vi "Digitizer Clock In Data.vi"(6 "Digitize Read Delay Ticks":u32, 9 "Digitize # Bits":u32=16, 10 "Convert Clock Ticks":u32=20, 11 "Refnum in":refnum<k21>) -> (3 "Data Out":T1 format="%.0x")   [LabVIEW 2017]
doc: "Author: Scott Hannahs <sth@magnet.fsu.edu>\nCopyright 2018 Florida State University, All rights reserved."
uses:
  <vilib>/eio/EIONode/EIONode.xnode
  <vilib>/rvi/eio/common/nirviEmuTemplateMethod_errors.vi
  SCH Data Controls/SCH Raw Int Data.ctl
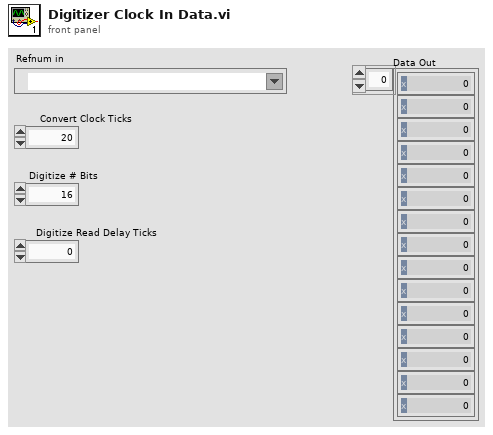
[diagram p1: front panel]
types:
  T1 = typedef "SCH Raw Int Data.ctl" = i16[]
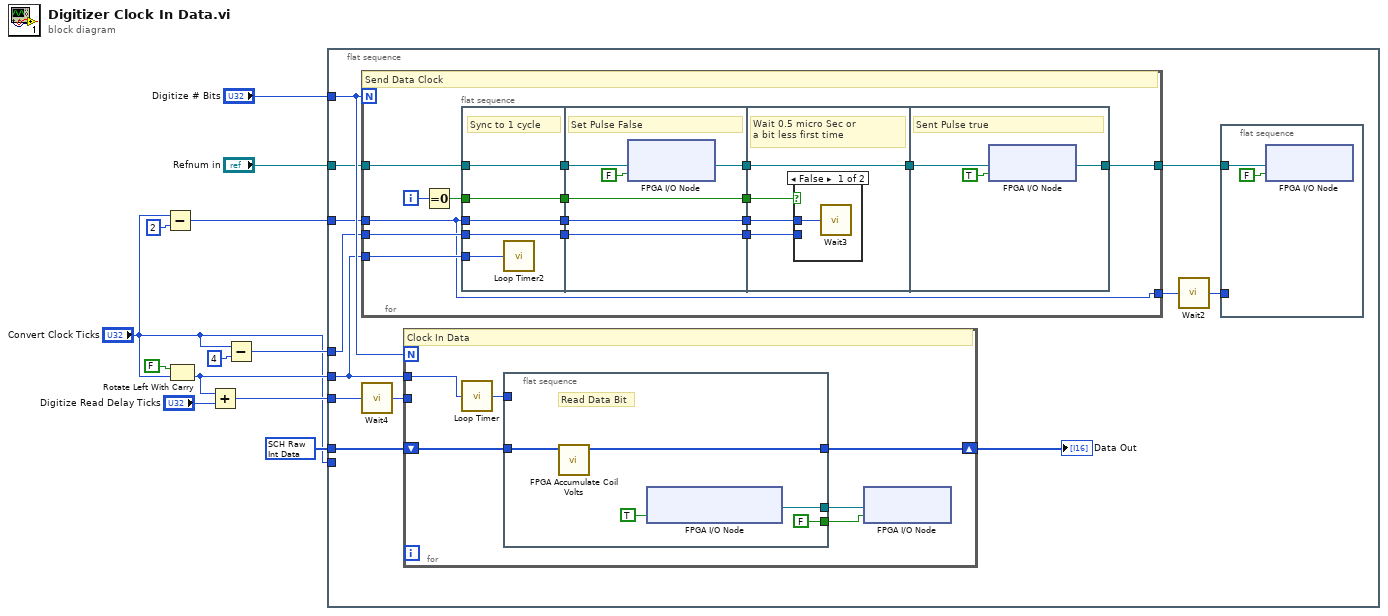
[diagram p0: block diagram]
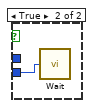
[diagram p2: hidden frame]
diagram:
  n1 = Subtract(x="Convert Clock Ticks", y=u32 2) -> (x-y=w1:u32)
  n2 = Rotate Left With Carry(2:"Convert Clock Ticks", 3:FALSE ("carry")) -> (0:w4:u32)  [unwired: 1 out]
  n3 = Add(x=w4, y="Digitize Read Delay Ticks") -> (x+y=w6:u32)
  n4 = Subtract(x="Convert Clock Ticks", y=u32 4) -> (x-y=w7:u32)
  n5 = flat-sequence {
    tunnel: "Digitize # Bits" -> [w24]
    tunnel: "Convert Clock Ticks" -> [_]
    tunnel: T1 [0, 0, 0, 0, 0, 0, 0, 0, 0, 0, 0, 0, 0, 0, 0, 0, 0, 0, 0, 0, 0, 0, 0, 0, 0, 0, 0, 0, 0, 0, 0, 0, 0, 0, 0, 0, 0, 0] -> [w22]
    tunnel: "Refnum in" -> [w21]
    tunnel: w4 -> [w20]
    tunnel: w7 -> [w19]
    tunnel: w6 -> [w18]
    tunnel: w1 -> [w17]
    frame #0 {
      n6 = for {
        N: w24 -> [_]
        tunnel: w21 -> [w42]
        tunnel: w20 -> [w39]
        tunnel: w19 -> [w37]
        tunnel: [w28] -> w15
        tunnel: [w27] -> w14
        tunnel: w17 -> [w27]
        i -> [w41]
        # "Send Data Clock"
        n7 = Equal To 0?(x=w41) -> (x = 0?=w38:bool)
        n8 = flat-sequence {
          tunnel: w37 -> [w44]
          tunnel: w38 -> [w45]
          tunnel: w39 -> [w43]
          tunnel: w27 -> [w46]
          tunnel: w42 -> [w47]
          tunnel: [w47] -> w36
          tunnel: [w46] -> w34
          tunnel: [w45] -> w32
          tunnel: [w44] -> w30
          tunnel: w36 -> [w50]
          tunnel: [w49] -> w35
          tunnel: w34 -> [w53]
          tunnel: [w53] -> w33
          tunnel: w32 -> [w52]
          tunnel: [w52] -> w31
          tunnel: w30 -> [w51]
          tunnel: [w51] -> w29
          tunnel: [w57] -> w40
          tunnel: w35 -> [w57]
          tunnel: w33 -> [w54]
          tunnel: w31 -> [w56]
          tunnel: w29 -> [w55]
          tunnel: w40 -> [w61]
          tunnel: [w60] -> w28
          frame #0 {
            # "Sync to 1 cycle"
            n9 = call "Loop Timer2"("Count(Ticks)"=w43) -> ()  [unwired: 1 out]
          }
          frame #1 {
            # "Set Pulse False"
            n10 = xnode "FPGA I/O Node"("I/O Item"=FALSE, "FPGA I/O In"=w50) -> ("FPGA I/O Out"=w49:refnum<k21>)  [unwired: 1 in, 1 out]
          }
          frame #2 {
            # "Wait 0.5 micro Sec or\na bit less first time"
            n11 = case shown="False" w56 {
              tunnel: w55 -> [_ w59]
              tunnel: w54 -> [w58 _]
              frame False {
                n12 = call "Wait3"("Count(Ticks)"=w58) -> ()  [unwired: 1 out]
              }
              frame True {
                n13 = call "Wait"("Count(Ticks)"=w59) -> ()  [unwired: 1 out]
              }
            }
          }
          frame #3 {
            # "Sent Pulse true"
            n14 = xnode "FPGA I/O Node"("I/O Item"=TRUE ("Connector0/DIO0"), "FPGA I/O In"=w61) -> ("FPGA I/O Out"=w60:refnum<k21>)
          }
        }
      }
      n15 = call "Wait4"("Count(Ticks)"=w18) -> ("Tick Count(Ticks)"=w23:u32)
      n16 = for {
        N: w24 -> [_]
        shift-right: [w68] -> w16
        shift-left: w22 -> [w67]
        tunnel: w23 -> [_]
        tunnel: w20 -> [w65]
        # "Clock In Data"
        n17 = call "Loop Timer"("Count(Ticks)"=w65) -> ("Tick Count(Ticks)"=w66:u32)
        n18 = flat-sequence {
          tunnel: [w73] -> w68
          tunnel: w67 -> [w72]
          tunnel: w66 -> [_]
          tunnel: [FALSE ("Digizer Data Read")] -> w64
          tunnel: [w69] -> w63
          frame #0 {
            # "Read Data Bit"
            n19 = call "FPGA Accumulate Coil Volts.vi"("Data Array In"=w72) -> ("Data Array Out"=w73:T1)  [unwired: 10 in]
            n20 = xnode "FPGA I/O Node"("Digizer Data Read"=TRUE) -> ("FPGA I/O Out"=w69:refnum<k21>)  [unwired: 1 in]
          }
        }
        n21 = xnode "FPGA I/O Node"("I/O Item"=w64, "FPGA I/O In"=w63) -> ()  [unwired: 1 out]
      }
      "Data Out" <- w16
      n22 = call "Wait2"("Count(Ticks)"=w14) -> ("Tick Count(Ticks)"=w13:u32)
      n23 = flat-sequence {
        tunnel: w15 -> [w26]
        tunnel: w13 -> [_]
        frame #0 {
          n24 = xnode "FPGA I/O Node"("I/O Item"=FALSE, "FPGA I/O In"=w26) -> ()  [unwired: 1 out]
        }
      }
    }
  }
